vi "XML_EEG_writeDataset.vi"(8 "error in (no error)":errorcluster, 9 "DatasetNumber":i32, 10 "XML_Dataset":T1, 11 "XML_EEG_File in":refnum<class "XML_EEG_File.lvclass">) -> (0 "error out":errorcluster, 2 "DOM document out":refnum<k20>, 3 "XML_EEG_File out":refnum<class "XML_EEG_File.lvclass">)   [LabVIEW 2016, in "XML_EEG_File_Parser.lvlib" / "XML_EEG_File.lvclass"]
uses:
  XML_EEG_File.lvclass
  XML_EEG_Dataset.ctl
  XML_EEG_File.lvclass/XML_EEG_File.ctl
  XML_EEG_timestampToHexString.vi
  XML_EEG_waveformToHexString.vi
  <vilib>/xml/NI_XML.lvlib
  <resource>/objmgr/DOMUserDefRef.rc
  XML_EEG_File_Parser.lvlib
panel:
  # "This VI is a part of BCI Design library, http://www.ru-bci.org \nCopyright © 2020, Sotnikov Peter, All rights reserved. License: GNU GPLv3"
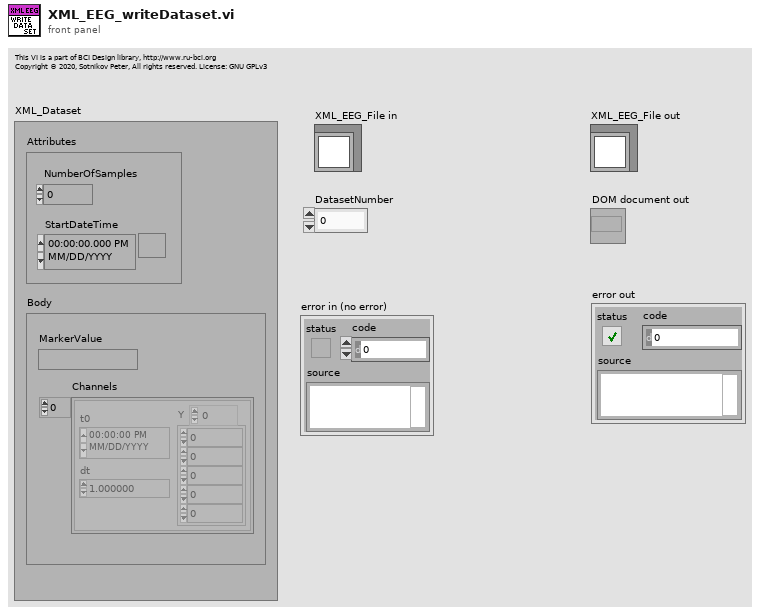
[diagram p1: front panel]
types:
  T1 = typedef "XML_EEG_File_Parser.lvlib/XML_EEG_Dataset.ctl" = cluster{"Attributes":cluster{"NumberOfSamples":i32, "StartDateTime":timestamp}, "Body":cluster{"MarkerValue":string, "Channels":waveform(dbl)[]}}
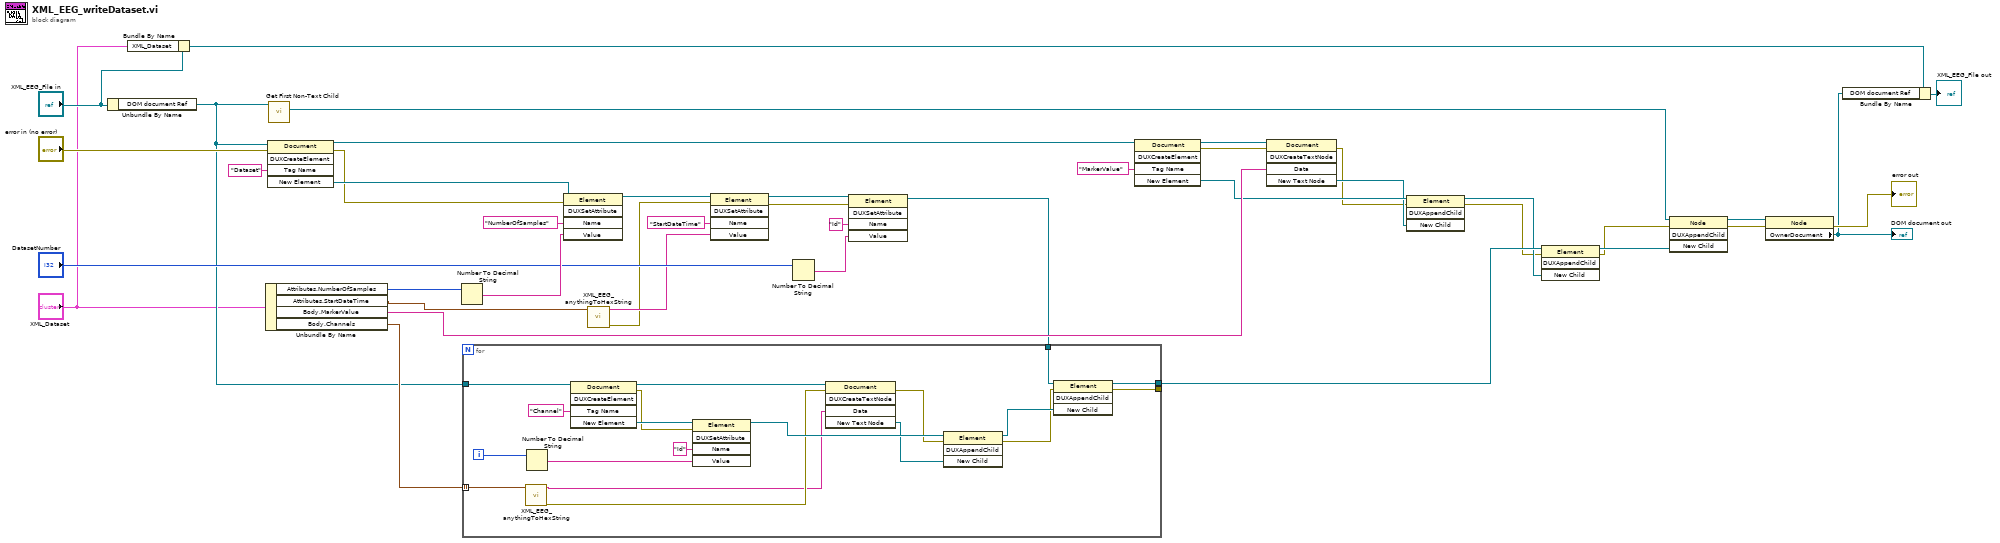
[diagram p0: block diagram]
diagram:
  n1 = Unbundle By Name("XML_EEG_File in") -> ("DOM document Ref"=w6:refnum<k20>)
  n2 = Bundle By Name(cluster="XML_EEG_File in", "XML_Dataset"="XML_Dataset") -> (w3:refnum<class "XML_EEG_File.lvclass">)
  n3 = Unbundle By Name("XML_Dataset") -> ("Attributes.NumberOfSamples"=w41:i32, "Attributes.StartDateTime"=w9:timestamp, "Body.MarkerValue"=w29:string, "Body.Channels"=w33:waveform(dbl)[])
  n4 = invoke class="Document" method="DUXCreateElement"(reference=w6, error in="error in (no error)", "Tag Name"="Dataset") -> (reference out=w32:refnum<k20>, error out=w37:errorcluster, "New Element"=w40:refnum<k20>)  [unwired: 2 in, 2 out]
  n5 = call <vilib>:"Get First Non-Text Child.vi"("node in"=w6) -> ("child node"=w20:refnum<k20>)  [unwired: 7 in, 3 out]
  n6 = Number To Decimal String(number=w41) -> (decimal integer string=w38:string)  [unwired: 1 in]
  n7 = invoke class="Element" method="DUXSetAttribute"(reference=w40, error in=w37, "Name"="NumberOfSamples", "Value"=w38) -> (reference out=w35:refnum<k20>)  [unwired: 1 in, 4 out]
  n8 = call-poly "XML_EEG_anythingToHexString.vi"("current time"=w9) -> ("error out"=w7:errorcluster, "HexString out"=w8:string)  [unwired: 9 in]
  n9 = invoke class="Element" method="DUXSetAttribute"(reference=w35, error in=w7, "Name"="StartDateTime", "Value"=w8) -> (reference out=w15:refnum<k20>, error out=w14:errorcluster)  [unwired: 1 in, 3 out]
  n10 = Number To Decimal String(number="DatasetNumber") -> (decimal integer string=w12:string)  [unwired: 1 in]
  n11 = invoke class="Element" method="DUXSetAttribute"(reference=w15, error in=w14, "Name"="Id", "Value"=w12) -> (reference out=w10:refnum<k20>)  [unwired: 1 in, 4 out]
  n12 = for {
    tunnel: w33 -> [w45] mode=indexing
    tunnel: w6 -> [w61]
    tunnel: [w48] -> w26
    tunnel: [w47] -> _
    tunnel: w10 -> [w46]
    i -> [w57]
    n13 = call-poly "XML_EEG_anythingToHexString.vi"("Analog waveform in"=w45) -> ("error out"=w44:errorcluster, "HexString out"=w43:string)  [unwired: 9 in]
    n14 = Number To Decimal String(number=w57) -> (decimal integer string=w56:string)  [unwired: 1 in]
    n15 = invoke class="Document" method="DUXCreateElement"(reference=w61, "Tag Name"="Channel") -> (reference out=w55:refnum<k20>, error out=w54:errorcluster, "New Element"=w59:refnum<k20>)  [unwired: 3 in, 2 out]
    n16 = invoke class="Element" method="DUXSetAttribute"(reference=w59, error in=w54, "Name"="Id", "Value"=w56) -> (reference out=w53:refnum<k20>)  [unwired: 1 in, 4 out]
    n17 = invoke class="Document" method="DUXCreateTextNode"(reference=w55, error in=w44, "Data"=w43) -> (error out=w51:errorcluster, "New Text Node"=w52:refnum<k20>)  [unwired: 2 in, 3 out]
    n18 = invoke class="Element" method="DUXAppendChild"(reference=w53, error in=w51, "New Child"=w52) -> (reference out=w50:refnum<k20>, error out=w49:errorcluster)  [unwired: 1 in, 2 out]
    n19 = invoke class="Element" method="DUXAppendChild"(reference=w46, error in=w49, "New Child"=w50) -> (reference out=w48:refnum<k20>, error out=w47:errorcluster)  [unwired: 1 in, 2 out]
  }
  n20 = invoke class="Document" method="DUXCreateElement"(reference=w32, "Tag Name"="MarkerValue") -> (reference out=w30:refnum<k20>, error out=w24:errorcluster, "New Element"=w28:refnum<k20>)  [unwired: 3 in, 2 out]
  n21 = invoke class="Document" method="DUXCreateTextNode"(reference=w30, error in=w24, "Data"=w29) -> (error out=w23:errorcluster, "New Text Node"=w27:refnum<k20>)  [unwired: 2 in, 3 out]
  n22 = invoke class="Element" method="DUXAppendChild"(reference=w28, error in=w23, "New Child"=w27) -> (reference out=w25:refnum<k20>, error out=w22:errorcluster)  [unwired: 1 in, 2 out]
  n23 = invoke class="Element" method="DUXAppendChild"(reference=w26, error in=w22, "New Child"=w25) -> (reference out=w21:refnum<k20>, error out=w18:errorcluster)  [unwired: 1 in, 2 out]
  n24 = invoke class="Node" method="DUXAppendChild"(reference=w20, error in=w18, "New Child"=w21) -> (reference out=w19:refnum<k20>, error out=w17:errorcluster)  [unwired: 1 in, 2 out]
  n25 = property class="Node"(reference=w19, error in=w17) -> (error out=→"error out":errorcluster, "OwnerDocument"=w2:refnum<k20>)  [unwired: 1 out]
  "DOM document out" <- w2
  n26 = Bundle By Name(cluster=w3, "DOM document Ref"=w2) -> (→"XML_EEG_File out":refnum<class "XML_EEG_File.lvclass">)
